vi "Handle Last Ack Core.vi"(4 "error in (no error)":errorcluster, 6 "Last Ack":refnum<class "Last Ack.lvclass">, 7 "AdvancedActor in":refnum<class "AdvancedActor.lvclass">) -> (0 "error out":errorcluster, 3 "AdvancedActor out":refnum<class "AdvancedActor.lvclass">)   [LabVIEW 2020, in "MGI-Panel Actor.lvlib" / "AdvancedActor.lvlib" / "AdvancedActor.lvclass"]
doc: "(<B>Filename</B>: Actor Framework.lvlib:Actor.lvclass:Handle Last Ack Core.vi)\n\nDefines how the caller actor responds to the Last Ack message from a nested actor. The Last Ack message is the final message a nested actor sends to its caller before it shuts down. The message contains information about the final state of the nested actor.\n\nBy default, this method does nothing except return any error the nested actor sent. A descendant class may override this method to define behavior."
uses:
  AdvancedActor.lvclass
  <vilib>/ActorFramework/LastAck/Last Ack.lvclass
  C:/Program Files (x86)/National Instruments/LabVIEW 2020/vi.lib/ActorFramework/Actor/Actor.lvclass
  <vilib>/Utility/error.llb/Error Cluster From Error Code.vi
  <vilib>/ActorFramework/Actor/Actor.lvclass
  <vilib>/ErrorRing/Error Ring.xnode
  D:/test/LabView_PanelManager/panel-actors/Source/AdvancedActor/AdvancedActor/AdvancedActor.lvclass
  D:/test/LabView_PanelManager/panel-actors/Source/AdvancedActor/AdvancedActorCaller/AdvancedActorCaller.lvclass
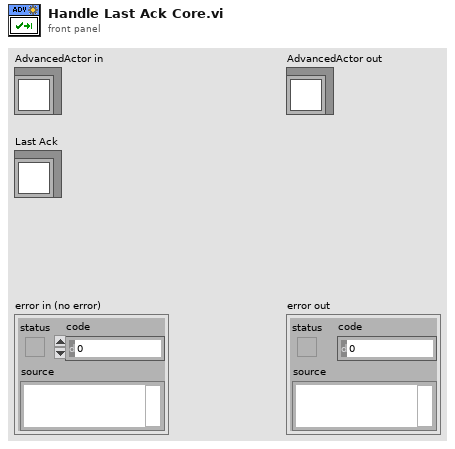
[diagram p1: front panel]
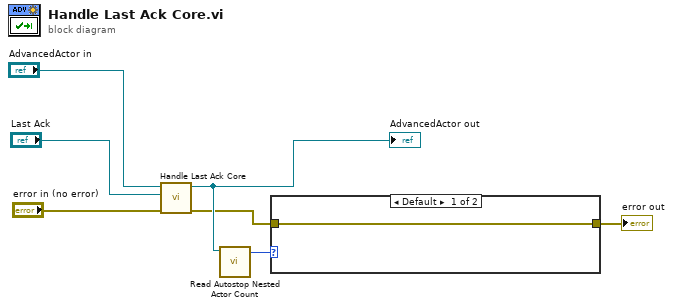
[diagram p0: block diagram]
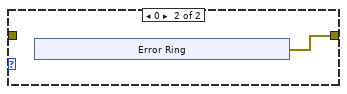
[diagram p2: hidden frame]
diagram:
  n1 = call-parent "Handle Last Ack Core.vi"("error in (no error)"="error in (no error)", "Last Ack"="Last Ack", "Actor in"="AdvancedActor in") -> ("error out"=w2:errorcluster, "Actor out"=w4:refnum<class "AdvancedActor.lvclass">)  [unwired: 3 in]
  "AdvancedActor out" <- w4
  n2 = call <vilib>:"Read Autostop Nested Actor Count.vi"("Actor in"=w4) -> ("Count"=w3:i32)  [unwired: 10 in]
  n3 = case shown="Default" w3 {
    tunnel: w2 -> [w8 _]
    tunnel: [w8 w9] -> w1
    frame Default {
    }
    frame 0 {
      n4 = xnode "Error Ring"() -> ("error out"=w9:errorcluster)
    }
  }
  "error out" <- w1
